vi "test Set Version.vi"(8 "error in (no error)":errorcluster, 11 "TestCase in":refnum<class "UUID Structure Tests.lvclass">) -> (0 "error out":errorcluster, 3 "TestCase out":refnum<class "UUID Structure Tests.lvclass">)   [LabVIEW 2015, in "UUID Structure Tests.lvclass"]
uses:
  UUID Structure Tests.lvclass
  <vilib>/addons/_JKI Toolkits/VI Tester/TestCase.llb/TestCase.lvclass
  UUID/UUID.lvclass
  <vilib>/Wiresmith Technology/VITAC (VI Tester Advanced Comparisons)/VITAC.lvlib
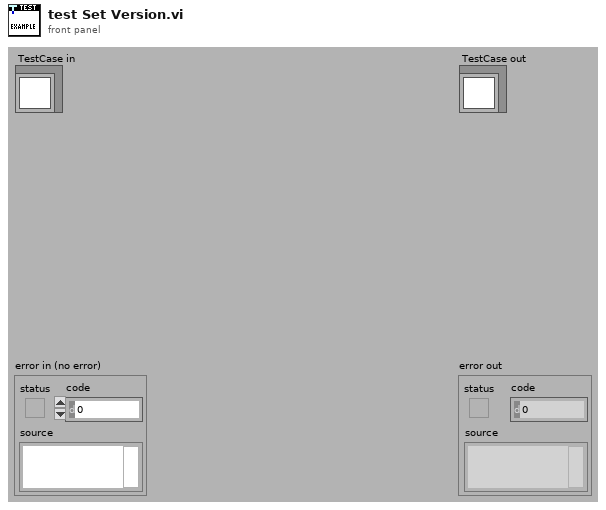
[diagram p1: front panel]
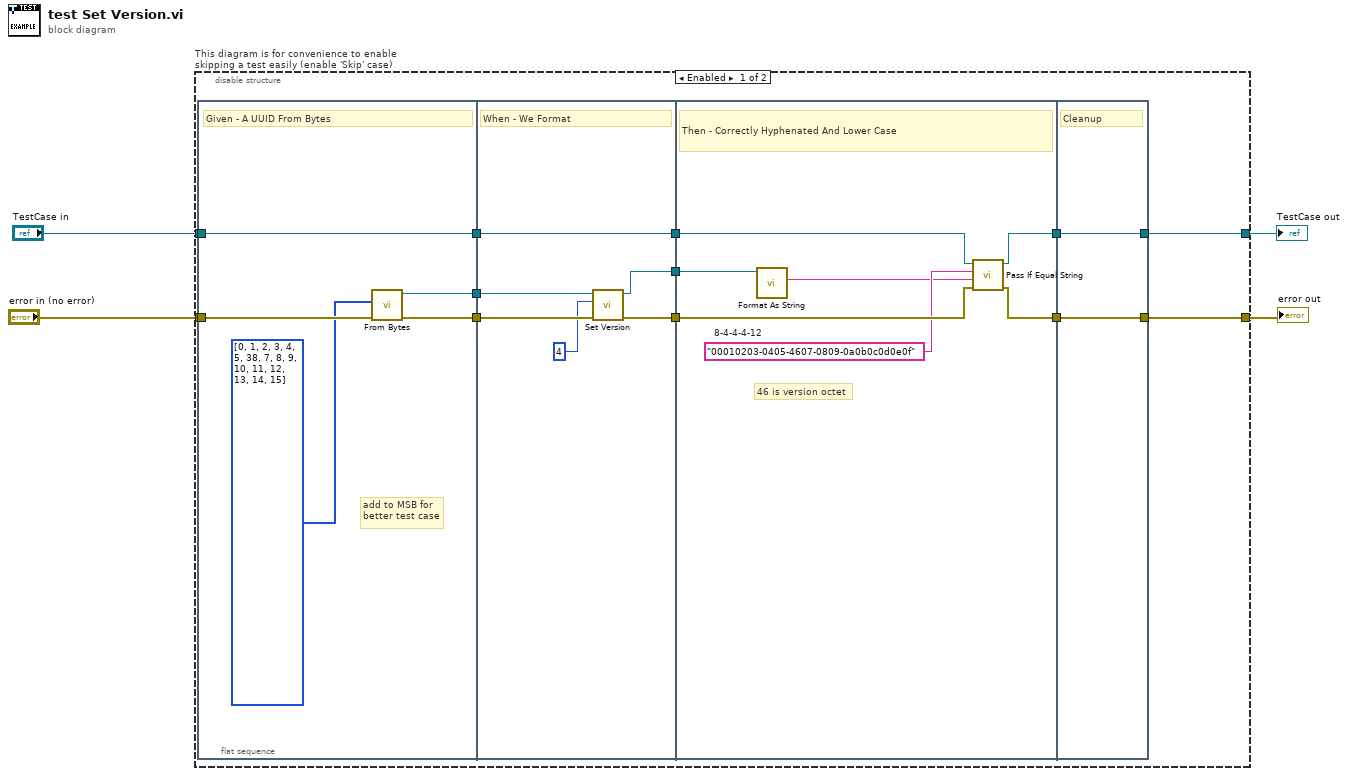
[diagram p0: block diagram]
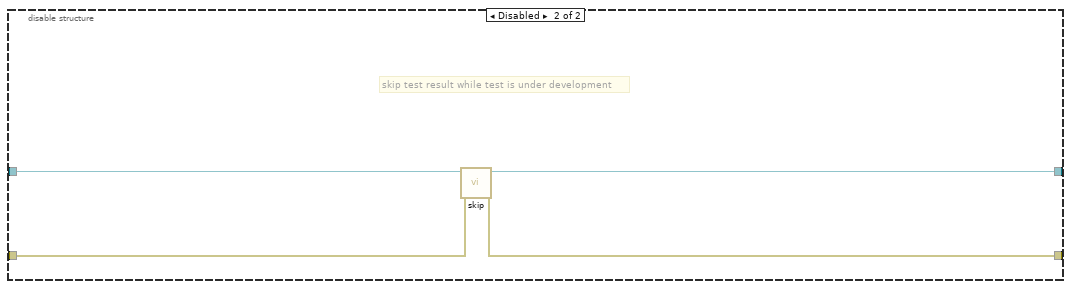
[diagram p2: hidden frame]
diagram:
  n1 = disable-structure "This diagram is for convenience to enable skipping a test easily (enable 'Skip' case)" shown="Enabled" {
    disable-tunnel: "TestCase in" -> [w10 w40]
    disable-tunnel: [w8 w38] -> w1
    disable-tunnel: [w7 w39] -> w3
    disable-tunnel: "error in (no error)" -> [w9 w37]
    frame Enabled {
      n2 = flat-sequence {
        tunnel: w9 -> [w20]
        tunnel: w10 -> [w21]
        tunnel: [w21] -> w16
        tunnel: [w19] -> w15
        tunnel: [w18] -> w6
        tunnel: [w27] -> w14
        tunnel: [w25] -> w13
        tunnel: w16 -> [w27]
        tunnel: w15 -> [w26]
        tunnel: w6 -> [w24]
        tunnel: [w23] -> w5
        tunnel: [w33] -> w12
        tunnel: [w31] -> w11
        tunnel: w14 -> [w34]
        tunnel: w13 -> [w32]
        tunnel: w5 -> [w29]
        tunnel: [w35] -> w7
        tunnel: [w36] -> w8
        tunnel: w12 -> [w36]
        tunnel: w11 -> [w35]
        frame #0 {
          # "add to MSB for\nbetter test case"
          # "Given - A UUID From Bytes"
          n3 = call "From Bytes.vi"("error in (no error)"=w20, "Bytes"=u8[] [0, 1, 2, 3, 4, 5, 38, 7, 8, 9, 10, 11, 12, 13, 14, 15]) -> ("error out"=w19:errorcluster, "UUID out"=w18:refnum<class "UUID.lvclass">)  [unwired: 8 in]
        }
        frame #1 {
          # "When - We Format"
          n4 = call "Set Version.vi"("error in (no error)"=w26, "Version"=u8 4, "UUID in"=w24) -> ("error out"=w25:errorcluster, "UUID out"=w23:refnum<class "UUID.lvclass">)  [unwired: 7 in]
        }
        frame #2 {
          w30 = "00010203-0405-4607-0809-0a0b0c0d0e0f"  # 8-4-4-4-12
          # "46 is version octet"
          # "Then - Correctly Hyphenated And Lower Case"
          n5 = call "Format As String.vi"("UUID.lvclass"=w29) -> ("String"=w28:string)  [unwired: 10 in]
          n6 = call <vilib>:"Pass If Equal String.vi"("error in (no error)"=w32, "actual"=w28, "expected"=w30, "TestCase in"=w34) -> ("error out"=w31:errorcluster, "TestCase out"=w33:refnum<class "UUID Structure Tests.lvclass">)  [unwired: 6 in]
        }
        frame #3 {
          # "Cleanup"
        }
      }
    }
    frame Disabled {
      # "skip test result while test is under development"
      n7 = call <vilib>:"skip.vi"("error in (no error)"=w37, "TestCase in"=w40) -> ("error out"=w39:errorcluster, "TestCase out"=w38:refnum<class "UUID Structure Tests.lvclass">)  [unwired: 8 in]
    }
  }
  "error out" <- w3
  "TestCase out" <- w1
